vi "Rotation toHuman player.vi"   [LabVIEW 2014]
uses:
  TypeDefs/SRE Enum.ctl
  <vilib>/Rock Robotics/Network Tables/SD Read Number.vi
  Support Code/Robot Global Data.vi
types:
  T1 = enum16{"High", "Middle", "Low", "Really Low", "Stopped"}
  T2 = typedef "SRE Enum.ctl" = enum16{"Start", "Run", "End"}
  T3 = cluster{"Speed":dbl, "Direction":dbl, "Rotation":dbl}
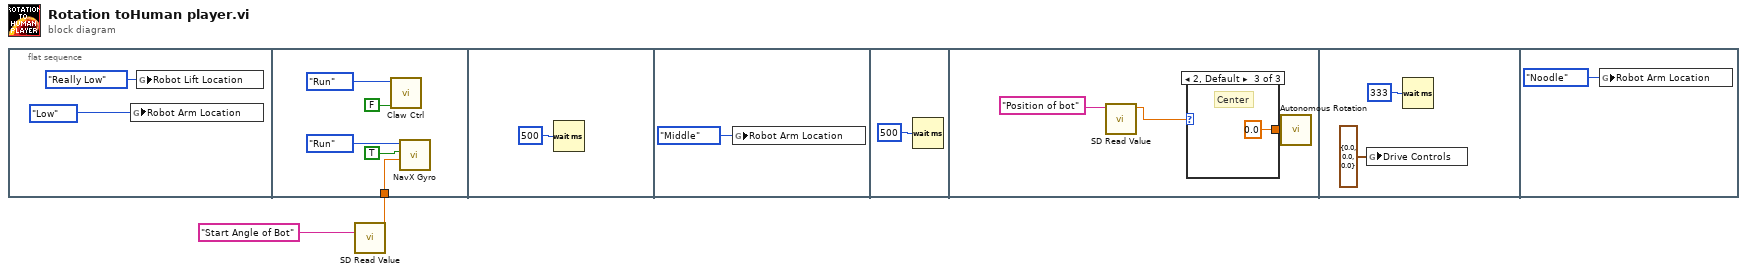
[diagram p0: block diagram]
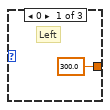
[diagram p2: hidden frame]
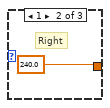
[diagram p3: hidden frame]
diagram:
  n1 = flat-sequence {
    tunnel: w1 -> [w5]
    frame #0 {
      n2 = global write "Robot Global Data.vi" "Robot Arm Location"(enum16{"High", "Middle", "Low", "Noodle"}."Low" ("Robot Arm Location")) -> ()
      n3 = global write "Robot Global Data.vi" "Robot Lift Location"(T1."Really Low" ("Robot Lift Location")) -> ()
    }
    frame #1 {
      n4 = call "Claw Ctrl.vi"("Open/Close"=FALSE, "Enum"=SRE_Enum."Run") -> ()  [unwired: 10 in]
      n5 = call "NavX Gyro.vi"("Set To"=w5, "Reset"=TRUE, "Enum"=SRE_Enum."Run") -> ()  [unwired: 7 in, 2 out]
    }
    frame #2 {
      n6 = Wait (ms)(milliseconds to wait=u32 500) -> ()  [unwired: 1 out]
    }
    frame #3 {
      n7 = global write "Robot Global Data.vi" "Robot Arm Location"(enum16{"High", "Middle", "Low", "Noodle"}."Middle" ("Robot Arm Location")) -> ()
    }
    frame #4 {
      n8 = Wait (ms)(milliseconds to wait=u32 500) -> ()  [unwired: 1 out]
    }
    frame #5 {
      n9 = call-poly <vilib>:"SD Read Value.vi"("Name"="Position of bot") -> ("Numeric"=w13:dbl)  [unwired: 8 in, 2 out]
      n10 = case shown="2, Default" w13 {
        tunnel: [300.0 ("Angle") 240.0 ("Angle") 0.0 ("Angle")] -> w15
        frame 0 {
          # "Left"
        }
        frame 1 {
          # "Right"
        }
        frame 2, Default {
          # "Center"
        }
      }
      n11 = call "Autonomous Rotation.vi"("Angle"=w15) -> ()  [unwired: 11 in]
    }
    frame #6 {
      n12 = global write "Robot Global Data.vi" "Drive Controls"(T3 {"Speed"=0.0, "Direction"=0.0, "Rotation"=0.0} ("Drive Controls")) -> ()
      n13 = Wait (ms)(milliseconds to wait=u32 333) -> ()  [unwired: 1 out]
    }
    frame #7 {
      n14 = global write "Robot Global Data.vi" "Robot Arm Location"(enum16{"High", "Middle", "Low", "Noodle"}."Noodle" ("Robot Arm Location")) -> ()
    }
  }
  n15 = call-poly <vilib>:"SD Read Value.vi"("Name"="Start Angle of Bot") -> ("Numeric"=w1:dbl)  [unwired: 8 in, 2 out]
